vi "To Msgpack.vi"(4 "Byte Array as Blobs":bool=TRUE, 6 "LabPack Shared Library":path=path "", 8 "Error In":errorcluster, 11 "Anything":variant) -> (0 "Error Out":errorcluster, 3 "Msgpack Data":u8[](array[numeric]))   [LabVIEW 2017, in "LabPack.lvlib"]
uses:
  LabPack.lvlib
  Writer/Private/Begin by Value.vi
  Writer/Private/End by Value.vi
  Writer/Writer.lvclass
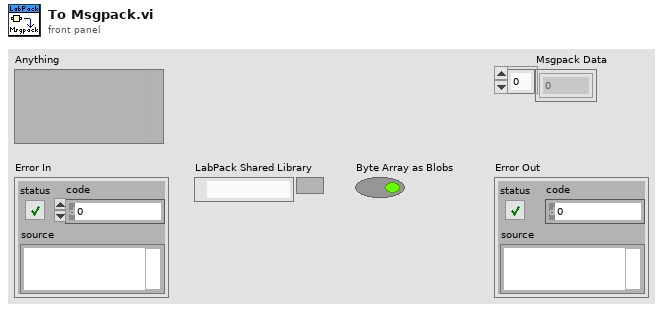
[diagram p1: front panel]
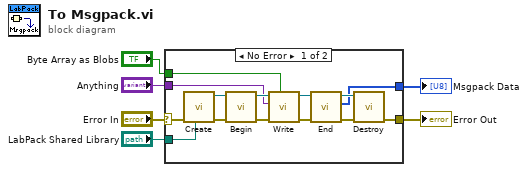
[diagram p0: block diagram]
diagram:
  n1 = case shown="No Error" "Error In" {
    selector: "Error In" -> [w20 w21]
    tunnel: [w16 w21] -> w5
    tunnel: "Anything" -> [w12 _]
    tunnel: [w8 _] -> w3
    tunnel: "Byte Array as Blobs" -> [w11 _]
    tunnel: "LabPack Shared Library" -> [w7 _]
    frame No Error {
      n2 = call "Create.vi"("LabPack Shared Library"=w7, "Error In"=w20) -> ("Error Out"=w19:errorcluster, "Writer"=w17:refnum<class "Writer.lvclass">)  [unwired: 8 in]
      n3 = call-poly "Begin.vi"("Error In"=w19, "Writer In"=w17) -> ("Error Out"=w18:errorcluster, "Writer Out"=w13:refnum<class "Writer.lvclass">)  [unwired: 8 in]
      n4 = call "Write.vi"("Byte Array as Blobs"=w11, "Error In"=w18, "Anything"=w12, "Writer In"=w13) -> ("Error Out"=w15:errorcluster, "Writer Out"=w14:refnum<class "Writer.lvclass">)  [unwired: 6 in]
      n5 = call-poly "End.vi"("Error In"=w15, "Writer In"=w14) -> ("Error Out"=w9:errorcluster, "Data"=w8:u8[], "Writer Out"=w10:refnum<class "Writer.lvclass">)  [unwired: 7 in]
      n6 = call "Destroy.vi"("Error In"=w9, "Writer"=w10) -> ("Error Out"=w16:errorcluster)  [unwired: 9 in]
    }
    frame Error {
    }
  }
  "Error Out" <- w5
  "Msgpack Data" <- w3
